vi "DotNETCam_Stop.vi"(8 "ErrorIn":errorcluster, 10 "CmdData":variant, 11 "DotNETCamIn":refnum<class>) -> (0 "ErrorOut":errorcluster, 2 "ReplyData":variant, 3 "DotNETCamOut":refnum<class>, 4 "Exit":bool)   [LabVIEW 2021, in "DotNETCam.lvclass"]
uses:
  DotNETCam.lvclass
  DotNETCam.lvclass/DotNETCam.ctl
  State.ctl
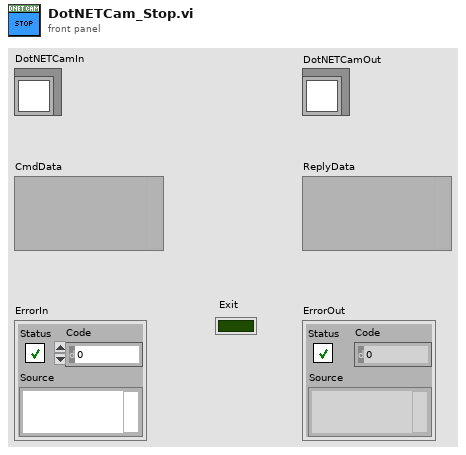
[diagram p1: front panel]
types:
  T1 = typedef "DotNETCam.lvclass/State.ctl" = enum16{"Idle", "Acquiring"}
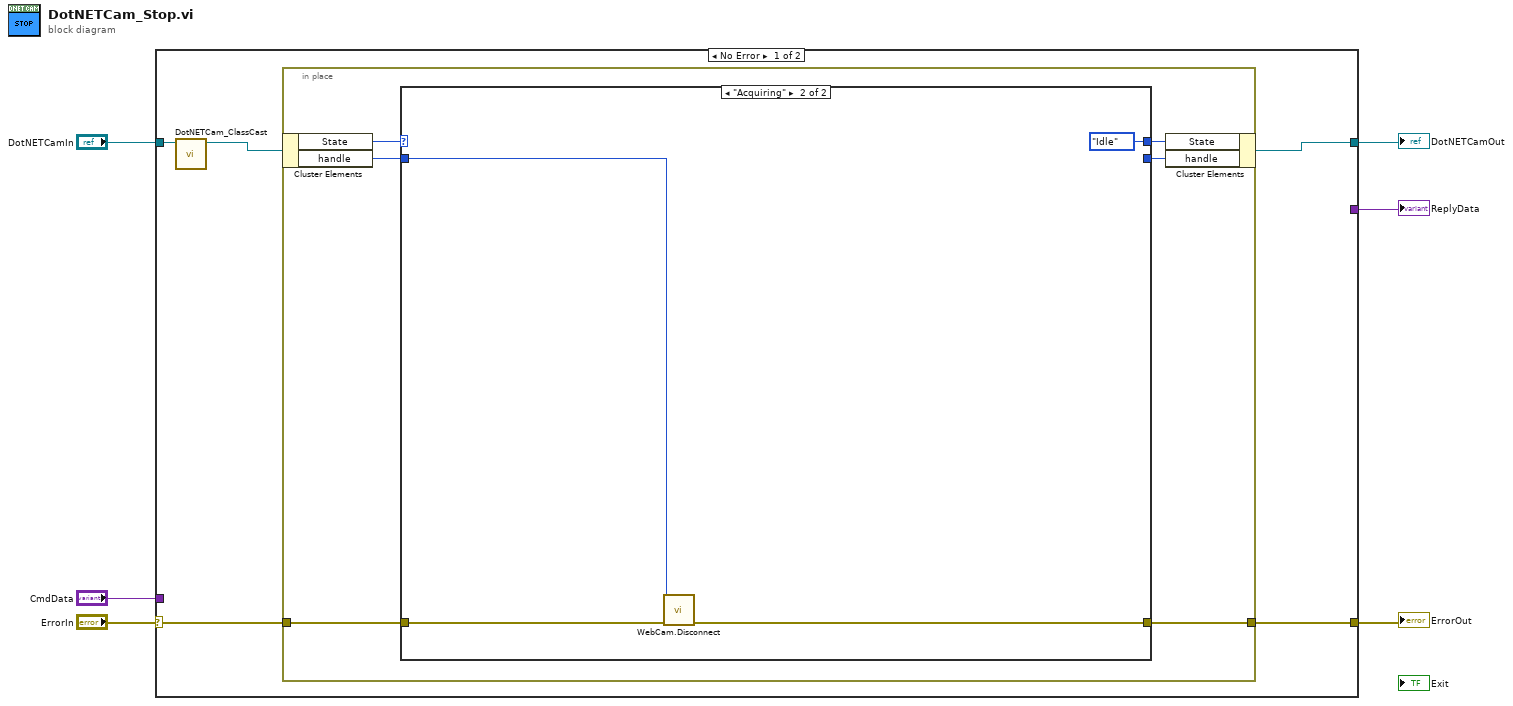
[diagram p0: block diagram]
diagram:
  n1 = case shown="No Error" "ErrorIn" {
    selector: "ErrorIn" -> [w11 w27]
    tunnel: [w10 w27] -> w5
    tunnel: [_ w26] -> w3
    tunnel: "CmdData" -> [_ w26]
    tunnel: "DotNETCamIn" -> [w9 w25]
    tunnel: [w7 w25] -> w1
    frame No Error {
      n2 = call "DotNETCam_ClassCast.vi"("DotNETCamIn"=w9) -> ("DotNETCamOut"=w8:refnum<class "DotNETCam.lvclass">)  [unwired: 10 in]
      n3 = in-place {
        in-place-border: w11 -> [w17]
        in-place-border: [w16] -> w10
        n4 = in-place-cluster #1(w8) -> ("State"=w15:T1, "handle"=w12:i32)
        n5 = case shown="\"Acquiring\"" w15 {
          selector: w15 -> [w19 _]
          tunnel: [w20 w23] -> w16
          tunnel: w17 -> [w20 w24]
          tunnel: [w19 State."Idle" ("State")] -> w14
          tunnel: [w18 _] -> w13
          tunnel: w12 -> [w18 w22]
          frame "Idle" {
          }
          frame "Acquiring" {
            n6 = call "WebCam.Disconnect.vi"("Handle"=w22, "ErrorIn"=w24) -> ("ErrorOut"=w23:errorcluster)  [unwired: 13 in]
          }
        }
        n7 = in-place-cluster #1("State"=w14, "handle"=w13) -> (w7:refnum<class "DotNETCam.lvclass">)
      }
    }
    frame Error {
    }
  }
  "ErrorOut" <- w5
  "DotNETCamOut" <- w1
  "ReplyData" <- w3
